vi "Undo.vi"(7 "Map Model in":refnum<class "Map Model.lvclass">, 8 "error in (no error)":errorcluster, 11 "Set Origin in":refnum<class "Set Origin.lvclass">) -> (0 "error out":errorcluster, 3 "Set Origin out":refnum<class "Set Origin.lvclass">, 5 "Map Model out":refnum<class "Map Model.lvclass">)   [LabVIEW 2020, in "Map Model.lvlib" / "Set Origin.lvclass"]
uses:
  Set Origin.lvclass
  Map Model/Map Model.lvclass
  Set Origin.lvclass/Set Origin.ctl
panel:
  # "NOTICE -- YOU MUST LEAVE THIS NOTICE IN PLACE.\n\nCopyright (c) 2017, LIANG LIU Shawn.Liu.cn@gmail.com\nAll rights reserved.\n\nRedistribution and use in source and binary forms, with or without modification, are permitted provided that the following conditions are met:\n-Redistributions of source code must retain the above copyright notice, this list of conditions and the following disclaimer.\n-Redistributions in binary form must reproduce the above copyright notice, this list of conditions and the following disclaimer in the documentation and/or other materials provided with the distribution.\n-Neither the name of the eLp nor the names of its contributors may be used to endorse or promote products derived from this software without specific prior written permission.\n\nTHIS SOFTWARE IS PROVIDED BY THE COPYRIGHT HOLDERS AND CONTRIBUTORS \"AS IS\" AND ANY EXPRESS OR IMPLIED WARRANTIES, INCLUDING, BUT NOT LIMITED TO, THE IMPLIED WARRANTIES OF MERCHANTABILITY AND FITNESS FOR A PARTICULAR PURPOSE ARE DISCLAIMED. IN NO EVENT SHALL THE COPYRIGHT HOLDER OR CONTRIBUTORS BE LIABLE FOR ANY DIRECT, INDIRECT, INCIDENTAL, SPECIAL, EXEMPLARY, OR CONSEQUENTIAL DAMAGES (INCLUDING, BUT NOT LIMITED TO, PROCUREMENT OF SUBSTITUTE GOODS OR SERVICES; LOSS OF USE, DATA, OR PROFITS; OR BUSINESS INTERRUPTION) HOWEVER CAUSED AND ON ANY THEORY OF LIABILITY, WHETHER IN CONTRACT, STRICT LIABILITY, OR TORT (INCLUDING NEGLIGENCE OR OTHERWISE) ARISING IN ANY WAY OUT OF THE USE OF THIS SOFTWARE, EVEN IF ADVISED OF THE POSSIBILITY OF SUCH DAMAGE."
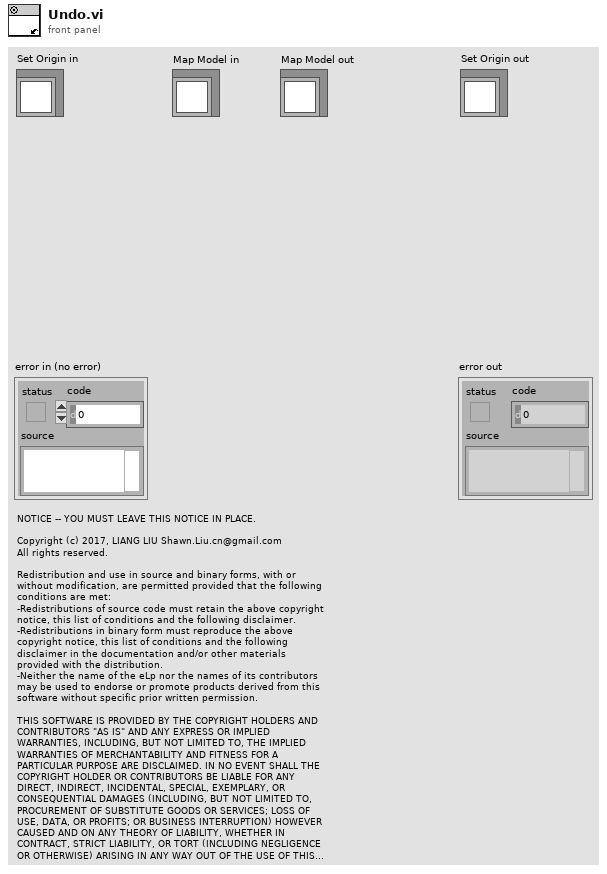
[diagram p1: front panel]
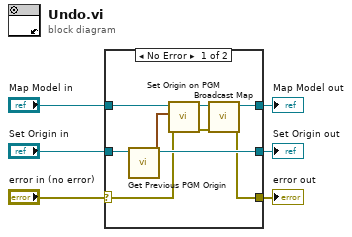
[diagram p0: block diagram]
diagram:
  n1 = case shown="No Error" "error in (no error)" {
    selector: "error in (no error)" -> [w8 w18]
    tunnel: "Map Model in" -> [w15 w17]
    tunnel: "Set Origin in" -> [w14 w16]
    tunnel: [w13 w16] -> w4
    tunnel: [w11 w17] -> w3
    tunnel: [w7 w18] -> w1
    frame No Error {
      n2 = call "Get Previous PGM Origin.vi"("Set Origin in"=w14) -> ("Previous PGM Origin"=w9:cluster{"Horizontal":dbl, "Vertical":dbl}, "Set Origin out"=w13:refnum<class "Set Origin.lvclass">)  [unwired: 9 in]
      n3 = call "Set Origin on PGM.vi"("error in (no error)"=w8, "Origin on PGM"=w9, "Map Model in"=w15) -> ("error out"=w10:errorcluster, "Map Model out"=w12:refnum<class "Map Model.lvclass">)  [unwired: 7 in]
      n4 = call "Broadcast Map.vi"("error in (no error)"=w10, "Map Model in"=w12) -> ("error out"=w7:errorcluster, "Map Model out"=w11:refnum<class "Map Model.lvclass">)  [unwired: 8 in]
    }
    frame Error {
    }
  }
  "error out" <- w1
  "Set Origin out" <- w4
  "Map Model out" <- w3
